vi "Send Error Msg.vi"(8 "error in":errorcluster, 11 "Qbus in":refnum<class "Qbus.lvclass">) -> (0 "error out":errorcluster, 3 "Qbus out":refnum<class "Qbus.lvclass">)   [LabVIEW 2021, in "EventLoggerProcess.lvlib"]
uses:
  EventLoggerProcess.lvlib
  <vilib>/addons/Qbus/Qbus.lvclass
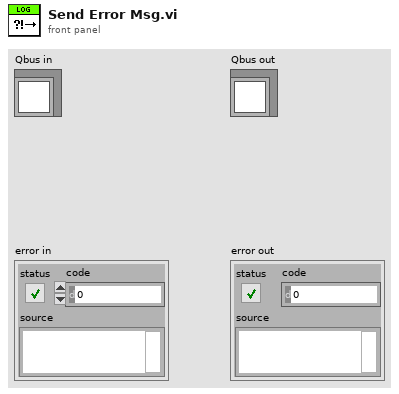
[diagram p1: front panel]
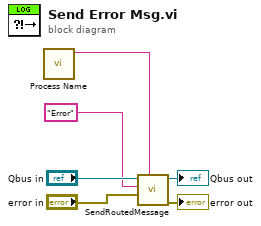
[diagram p0: block diagram]
diagram:
  n1 = call "Process Name.vi"() -> ("process name"=w3:string)  [unwired: 11 in]
  n2 = call <vilib>:"SendRoutedMessage.vi"("listener process"=w3, "message value"="error in", "message name"="Error", "Qbus in"="Qbus in") -> ("error in (no error)"=→"error out":errorcluster, "Qbus out"=→"Qbus out":refnum<class "Qbus.lvclass">)  [unwired: 6 in]
